vi "T7 Stream Enable KAG.vi"(0 "IP Configuration":T1={"Connection ID In"=refnum, "Connection ID Out"=refnum, "Device IP"="192.168.126.147", "Port"=502}, 5 "Enable":enum32{"Disable", "Enable"}(ring), 11 "error in":errorcluster) -> (15 "error out":errorcluster)   [LabVIEW 2015]
doc: "Write Stream ENABLE LabJack Register via MODBUS."
uses:
  T7 IP Config KAG.ctl
  T7Examples/MODBUS/T7MOD_Read_UINT32_Register.vi
  T7Examples/MODBUS/T7MOD_Write_UINT32_Register.vi
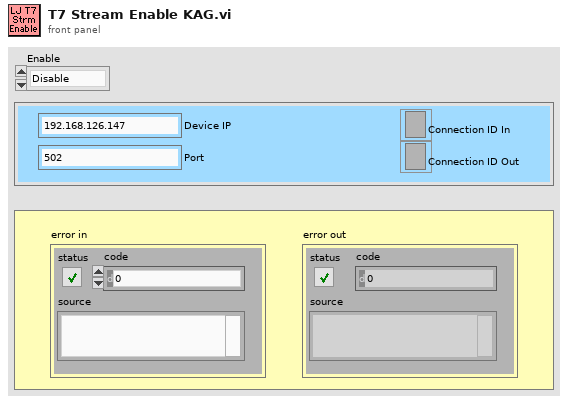
[diagram p1: front panel]
types:
  T1 = typedef "T7 IP Config KAG.ctl" = cluster{"Connection ID In":refnum<k5>, "Connection ID Out":refnum<k5>, "Device IP":string, "Port":i32}
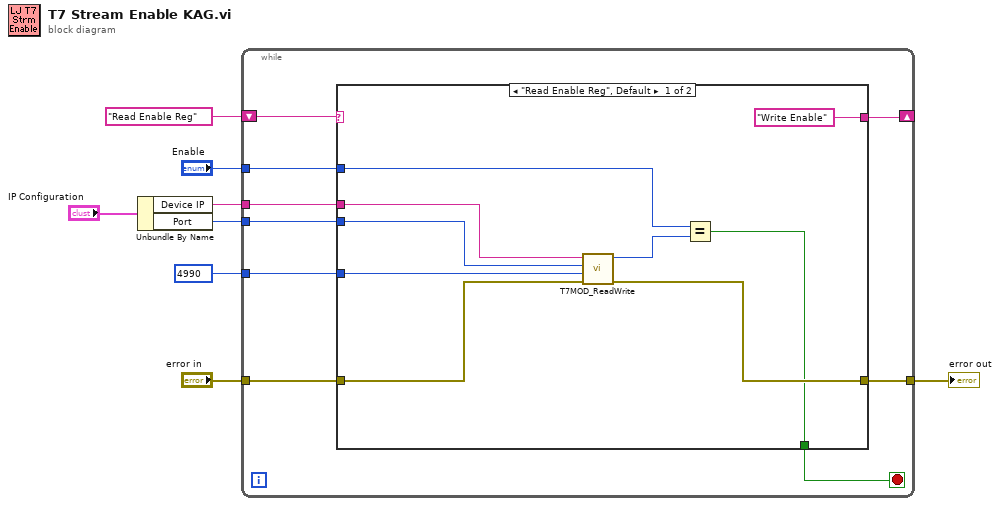
[diagram p0: block diagram]
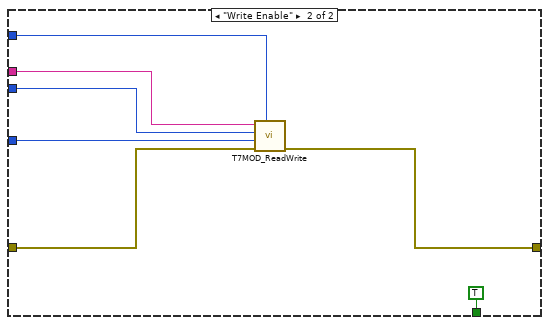
[diagram p2: hidden frame]
diagram:
  n1 = Unbundle By Name("IP Configuration") -> ("Device IP"=w4:string, "Port"=w3:i32)
  n2 = while {
    shift-right: [w16] -> _
    shift-left: "Read Enable Reg" -> [w17]
    tunnel: "error in" -> [w15]
    tunnel: [w14] -> w5
    tunnel: w4 -> [w13]
    tunnel: w3 -> [w12]
    tunnel: "Enable" -> [w11]
    tunnel: 4990 ("LabJack UINT32 Register") -> [w10]
    stop <- w9 stop-if-true
    n3 = case shown="\"Read Enable Reg\", Default" w17 {
      tunnel: ["Write Enable" _] -> w16
      tunnel: w15 -> [w25 w33]
      tunnel: [w24 w32] -> w14
      tunnel: w13 -> [w23 w31]
      tunnel: w12 -> [w22 w30]
      tunnel: w11 -> [w21 w28]
      tunnel: w10 -> [w19 w29]
      tunnel: [w18 TRUE] -> w9
      frame "Read Enable Reg", Default {
        n4 = call-poly "T7MOD_ReadWrite.vi"("error in"=w25, "LabJack UINT32 Register"=w19, "Remote Port"=w22, "Remote IP Address"=w23) -> ("error out"=w24:errorcluster, "Read UINT32"=w20:u32)  [unwired: 4 in, 2 out]
        n5 = Equal?(x=w21, y=w20) -> (x = y?=w18:bool)
      }
      frame "Write Enable" {
        n6 = call-poly "T7MOD_ReadWrite.vi"("UINT32 to Write"=w28, "error in"=w33, "LabJack UINT32 Register"=w29, "Remote Port"=w30, "Remote IP Address"=w31) -> ("error out"=w32:errorcluster)  [unwired: 5 in, 1 out]
      }
    }
  }
  "error out" <- w5
